vi "get_price.vi"(8 "error in (no error)":errorcluster, 11 "IFurniture in":refnum<class "IFurniture.lvclass">) -> (0 "error out":errorcluster, 2 "price":dbl, 3 "IFurniture out":refnum<class "IFurniture.lvclass">)   [LabVIEW 2024, in "IFurniture.lvclass"]
uses:
  IFurniture.lvclass
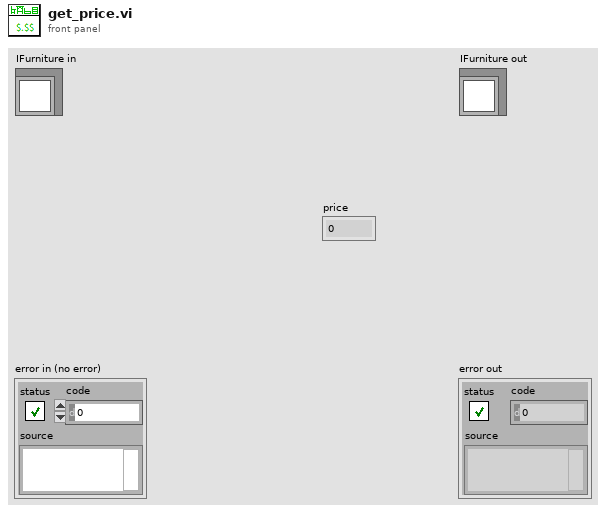
[diagram p1: front panel]
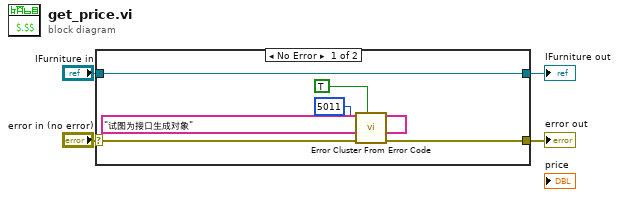
[diagram p0: block diagram]
diagram:
  n1 = case shown="No Error" "error in (no error)" {
    selector: "error in (no error)" -> [w7 w12]
    tunnel: [w6 w12] -> w3
    tunnel: [w10 w11] -> w1
    tunnel: "IFurniture in" -> [w10 w11]
    frame No Error {
      n2 = call <vilib>:"Error Cluster From Error Code.vi"("show call chain? (False)"=TRUE, "error in (no error)"=w7, "error message (\"\")"="试图为接口生成对象" ("error message (\"\")"), "error code (0)"=5011) -> ("error out"=w6:errorcluster)  [unwired: 5 in]
    }
    frame Error {
    }
  }
  "error out" <- w3
  "IFurniture out" <- w1
